vi "monitor_quspin_input.vi"(6 "Cluster":T2, 9 "Cluster 2":T2, 10 "Controls[]":refnum<vi>[](array[refnum]), 11 "VISA Refnum in":refnum<visa-resource-name>) -> ()   [LabVIEW 2015]
uses:
  Control 1.ctl
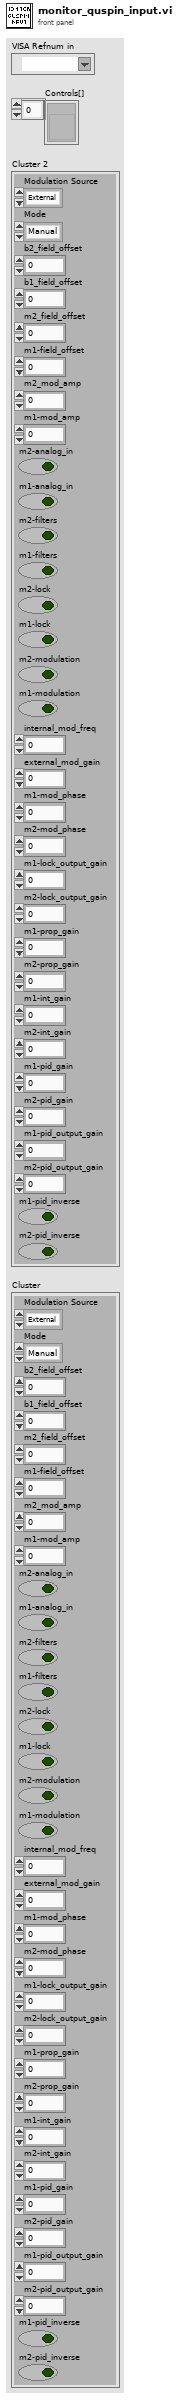
[diagram p1: front panel]
types:
  T1 = typedef "Control 1.ctl" = dbl
  T2 = cluster{"Modulation Source":enum32{"External", "Internal"}, "Mode":enum32{"Manual", "TTL"}, "b2_field_offset":dbl, "b1_field_offset":dbl, "m2_field_offset":dbl, "m1-field_offset":dbl, "m2_mod_amp":dbl, "m1-mod_amp":dbl, "m2-analog_in":bool, "m1-analog_in":bool, "m2-filters":bool, "m1-filters":bool, "m2-lock":bool, "m1-lock":bool, "m2-modulation":bool, "m1-modulation":bool, "internal_mod_freq":dbl, "external_mod_gain":dbl, "m1-mod_phase":T1, "m2-mod_phase":dbl, "m1-lock_output_gain":dbl, "m2-lock_output_gain":dbl, "m1-prop_gain":dbl, "m2-prop_gain":dbl, "m1-int_gain":dbl, "m2-int_gain":dbl, "m1-pid_gain":dbl, "m2-pid_gain":dbl, "m1-pid_output_gain":dbl, "m2-pid_output_gain":dbl, "m1-pid_inverse":bool, "m2-pid_inverse":bool}
  T3 = cluster{"Modulation Source":bool, "Mode":bool, "b2_field_offset":bool, "b1_field_offset":bool, "m2_field_offset":bool, "m1-field_offset":bool, "m2_mod_amp":bool, "m1-mod_amp":bool, "m2-analog_in":bool, "m1-analog_in":bool, "m2-filters":bool, "m1-filters":bool, "m2-lock":bool, "m1-lock":bool, "m2-modulation":bool, "m1-modulation":bool, "internal_mod_freq":bool, "external_mod_gain":bool, "m1-mod_phase":bool, "m2-mod_phase":bool, "m1-lock_output_gain":bool, "m2-lock_output_gain":bool, "m1-prop_gain":bool, "m2-prop_gain":bool, "m1-int_gain":bool, "m2-int_gain":bool, "m1-pid_gain":bool, "m2-pid_gain":bool, "m1-pid_output_gain":bool, "m2-pid_output_gain":bool, "m1-pid_inverse":bool, "m2-pid_inverse":bool}
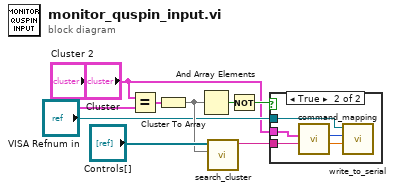
[diagram p0: block diagram]
diagram:
  n1 = Equal?(x="Cluster", y="Cluster 2") -> (x = y?=w4:T3)
  n2 = Cluster To Array(cluster=w4) -> (array=w6:bool[])
  n3 = And Array Elements(Boolean array=w6) -> (logical AND=w2:bool)
  n4 = call "search_cluster.vi"("change?"=w6, "Controls[]"="Controls[]") -> ("Label.Text"=w8:string)  [unwired: 9 in]
  n5 = Not(x=w2) -> (.not. x?=w9:bool)
  n6 = case shown="True" w9 {
    tunnel: "Cluster" -> [_ w13]
    tunnel: w8 -> [_ w14]
    tunnel: "VISA Refnum in" -> [_ w12]
    frame False {
    }
    frame True {
      n7 = call "command_mapping.vi"("Cluster"=w13, "cmd in"=w14) -> ("address out"=w11:i16, "value out"=w10:T1)  [unwired: 7 in]
      n8 = call "write_to_serial.vi"("value in"=w10, "address in"=w11, "VISA Refnum in"=w12) -> ()  [unwired: 9 in]
    }
  }
